vi "alphanumkey_user.vi"(11 "String 2":string) -> (1 "OK?":bool, 3 "String":string)   [LabVIEW 2014]
panel:
  out "error constant":errorcluster
  in  "Cancel Button":bool
  in  "OK Button":bool
  in  "Boolean":bool
  in  "Shift 4":bool
  in  "Shift 3":bool
  in  "H 31":bool
  in  "H 30":bool
  in  "H 29":bool
  in  "H 28":bool
  in  "H 27":bool
  in  "H 26":bool
  in  "H 25":bool
  in  "H 24":bool
  in  "H 23":bool
  in  "H 22":bool
  in  "H 21":bool
  in  "H 20":bool
  in  "Shift 2":bool
  in  "H 19":bool
  in  "H 18":bool
  in  "H 17":bool
  in  "H 16":bool
  in  "H 15":bool
  in  "H 14":bool
  in  "H 13":bool
  in  "H 12":bool
  in  "H 11":bool
  in  "H 10":bool
  in  "H 9":bool
  in  "H 8":bool
  in  "H 7":bool
  in  "H 6":bool
  in  "H 5":bool
  in  "H 4":bool
  in  "H 3":bool
  in  "H 2":bool
  in  "H":bool
  in  "G":bool
  in  "F":bool
  in  "E":bool
  in  "D":bool
  in  "C":bool
  in  "B":bool
  in  "Shift":bool
  in  "A":bool
  in  "Blank Button":bool
  in  "stop":bool
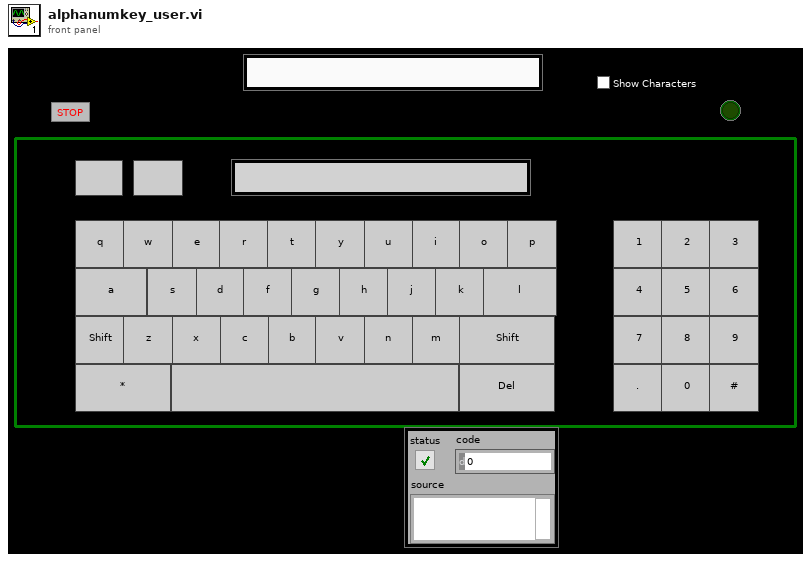
[diagram p1: front panel]
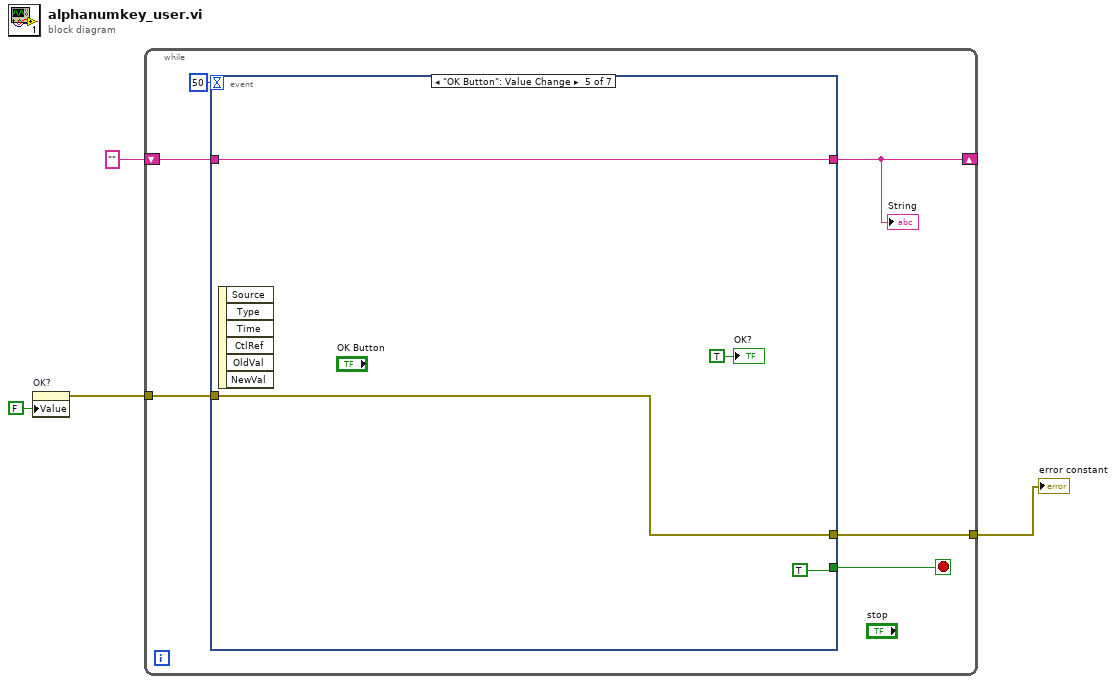
[diagram p0: block diagram]
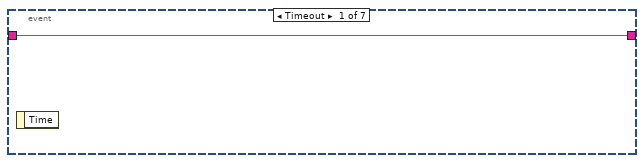
[diagram p2: hidden frame]
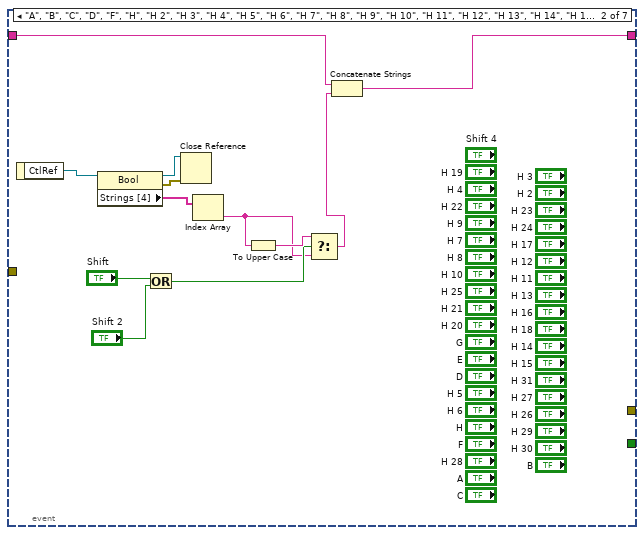
[diagram p3: hidden frame]
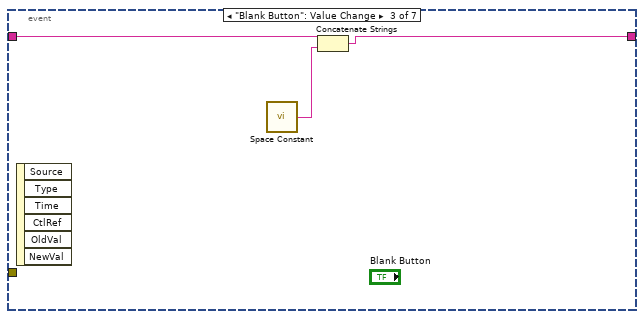
[diagram p4: hidden frame]
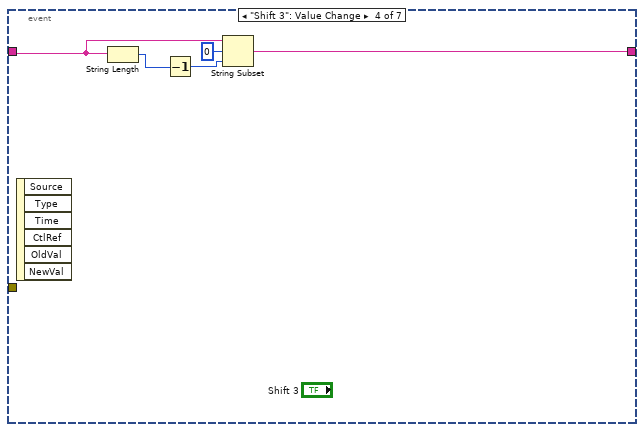
[diagram p5: hidden frame]
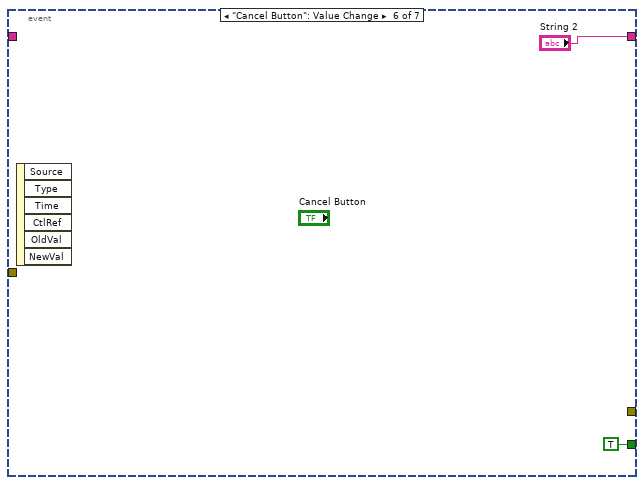
[diagram p6: hidden frame]
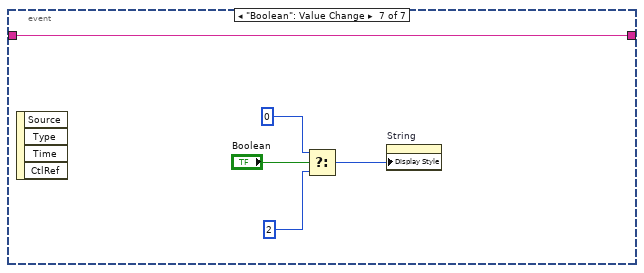
[diagram p7: hidden frame]
diagram:
  n1 = property on="OK?" class="Bool (strict)"("Value"=FALSE ("OK?")) -> (error out=w1:errorcluster)  [unwired: 2 in, 1 out]
  n2 = while {
    shift-right: [w9] -> _
    shift-left: "" ("String 2") -> [w8]
    tunnel: [w6] -> w2
    tunnel: w1 -> [w5]
    stop <- w7 stop-if-true
    n3 = event shown="[4] \"OK Button\": Value Change" {
      selector: _ -> [_ _ _ _ _ _ _]
      dyn-events: _ -> [_ _ _ _ _ _ _]
      timeout: 50 -> [_ _ _ _ _ _ _]
      tunnel: [w11 w18 w24 w27 w35 "String 2" w38] -> w9
      tunnel: w8 -> [w11 w19 w26 w31 w35 _ w38]
      tunnel: [_ _ _ _ TRUE TRUE _] -> w7
      tunnel: [_ _ _ _ w32 _ _] -> w6
      tunnel: w5 -> [_ _ _ _ w32 _ _]
      event Timeout {
        n4 = event-data() -> ()  [unwired: 1 in, 1 out]
      }
      event "A", "B", "C", "D", "F", "H", "H 2", "H 3", "H 4", "H 5", "H 6", "H 7", "H 8", "H 9", "H 10", "H 11", "H 12", "H 13", "H 14", "H 15", "H 16", "H 17", "H 18", "H 19", "H 20", "H 21", "H 22", "H 23", "H 24", "H 25", "H 26", "H 27", "H 28", "H 29", "H 30", "H 31", "E", "G", "Shift 4": Value Change {
        n5 = event-data() -> ("CtlRef"=w23:refnum<vi>)  [unwired: 1 in]
        n6 = property class="Bool"(reference=w23) -> (reference out=w21:refnum<vi>, error out=w20:errorcluster, "Strings [4]"=w22:string[])  [unwired: 1 in]
        n7 = Or(x="Shift", y="Shift 2") -> (x .or. y?=w13:bool)
        n8 = Close Reference(reference=w21, error in (no error)=w20) -> ()  [unwired: 1 out]
        n9 = Index Array(array=w22) -> (element=w12:string)  [unwired: 1 in]
        n10 = To Upper Case(1:w12) -> (0:w17:string)
        n11 = Select(t=w17, s=w13, f=w12) -> (s? t:f=w16:string)
        n12 = Concatenate Strings(w19, w16) -> (w18:string)
      }
      event "Blank Button": Value Change {
        n13 = event-data() -> ()  [unwired: 1 in, 6 out]
        n14 = call <vilib>:"Space Constant.vi"() -> ("String"=w25:string)
        n15 = Concatenate Strings(w26, w25) -> (w24:string)
      }
      event "Shift 3": Value Change {
        n16 = event-data() -> ()  [unwired: 1 in, 6 out]
        n17 = String Length(string=w31) -> (length=w29:i32)
        n18 = Decrement(x=w29) -> (x-1=w28:i32)
        n19 = String Subset(string=w31, offset (0)=0, length (rest)=w28) -> (substring=w27:string)
      }
      event "OK Button": Value Change {
        n20 = event-data() -> ()  [unwired: 1 in, 6 out]
        "OK?" <- TRUE ("OK?")
      }
      event "Cancel Button": Value Change {
        n21 = event-data() -> ()  [unwired: 1 in, 6 out]
      }
      event "Boolean": Value Change {
        n22 = event-data() -> ()  [unwired: 1 in, 4 out]
        n23 = Select(t=u32 0, s="Boolean", f=u32 2) -> (s? t:f=w39:u32)
        n24 = property on="String" class="Str"("Display Style"=w39) -> ()  [unwired: 2 in, 2 out]
      }
    }
    "String" <- w9
  }
  "error constant" <- w2
